vi "Construct TCP Connection.vi"(7 "ID":string, 9 "Read Mode (Standard)":T1(ring), 10 "Write Timeout (25000 ms)":i32=25000, 11 "ConnectionRef":refnum<k5>) -> (3 "TCP Connection out":refnum<class "TCP Connection.lvclass">)   [LabVIEW 2017, in "TCP Interface.lvlib" / "TCP Connection.lvclass"]
uses:
  <vilib>/gpm_packages/@cs/Network-sink/Source/TCP Interface/TCP Connection/TCP Connection.lvclass
  C:/Program Files/National Instruments/LabVIEW 2017/vi.lib/gpm_packages/@cs/Network-sink/Source/Network Interface/IConnection/IConnection.lvclass
  <vilib>/gpm_packages/@cs/Network-sink/Source/TCP Interface/TCP Connection/TCP Connection.lvclass/TCP Connection.ctl
  <vilib>/gpm_packages/@cs/Network-sink/Source/Network Interface/IConnection/IConnection.lvclass/IConnection.ctl
  <vilib>/gpm_packages/@cs/Network-sink/Source/Network Interface/IConnection/IConnection.lvclass
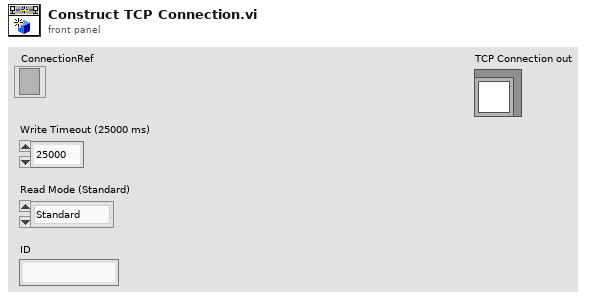
[diagram p1: front panel]
types:
  T1 = enum16{"Standard", "Buffered", "CRLF", "Immediate"}
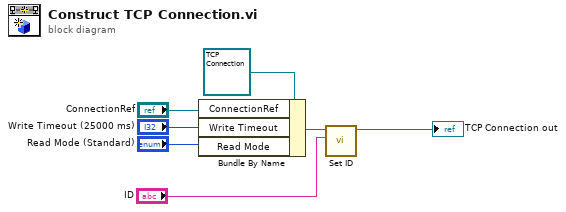
[diagram p0: block diagram]
diagram:
  n1 = Bundle By Name(cluster=refnum<class "TCP Connection.lvclass"> refnum ("TCP Connection in"), "ConnectionRef"="ConnectionRef", "Write Timeout"="Write Timeout (25000 ms)", "Read Mode"="Read Mode (Standard)") -> (w3:refnum<class "TCP Connection.lvclass">)
  n2 = call <vilib>:"Set ID.vi"("ID"="ID", "IConnection in"=w3) -> ("IConnection out"=→"TCP Connection out":refnum<class "TCP Connection.lvclass">)  [unwired: 9 in]
